vi "GenesysPS.destructor.vi"(0 "i ref in":refnum<vi>, 5 "error in (no error)":errorcluster) -> (19 "error out":errorcluster)   [LabVIEW 2014, in "GenesysPS.lvlib"]
doc: "This is the destructor of a class.\n\nLicense Agreement for this software:\n\nCopyright (C)\nGesellschaft für Schwerionenforschung, GSI\nPlanckstr. 1\n64291 Darmstadt\nGermany\n\nContact: D.Beck@gsi.de \n\nThis program is free software; you can redistribute it and/or modify it under the terms of the \nGNU General Public License as published by the Free Software Foundation; either version 2 of \nthe license, or (at your option) any later version.\n\nThis program is distributed in the hope that it will be useful, but WITHOUT ANY WARRANTY; \nwithout even the implied warranty of MERCHANTABILITY or FITNESS FOR A PARTICULAR PURPOSE. See the GNU General License for more details (http://www.gnu.org).\n\nGesellschaft für Schwerionenforschung, GSI\nPlanckstr. 1, 64291 Darmstadt, Germany\nFor all questions and ideas contact: M.Richter@gsi.de, H.Brand@gsi.de or D.Beck@gsi.de.\nLast update: 16-JUN-2004"
uses:
  GenesysPS.lvlib
  DIMPowerSupply/DIMPowerSupply.lvlib
  CSlibraries-extern/DimLVEvent/LVDimInterface/LVDimInterface.lvlib
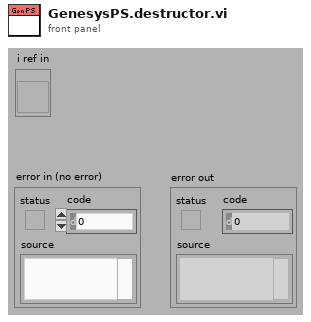
[diagram p1: front panel]
types:
  T1 = typedef "GenesysPS.lvlib/GenesysPS.i attribute.ctl" = cluster{"VISA name/ Heizinger":refnum<visa-resource-name>, "GEN Addr":i32, "WithTempInt?":bool, "TempLimit":dbl, "TemperatureID":i32, "Temp queue":refnum<queue>}
  T2 = enum16{"SetAttribute", "GetAttribute", "CreateAttribute", "DestroyAttribute", "DestroyAllAtributes"}
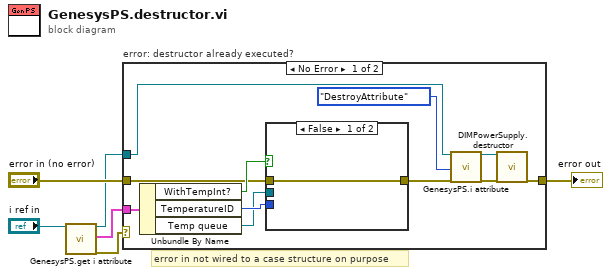
[diagram p0: block diagram]
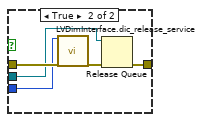
[diagram p2: hidden frame]
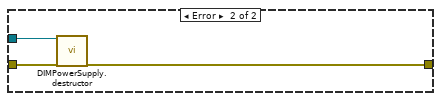
[diagram p3: hidden frame]
diagram:
  # "error in not wired to a case structure on purpose"
  n1 = call "GenesysPS.get i attribute.vi"("i ref in"="i ref in") -> ("i ref out"=w2:refnum<vi>, "i attribute"=w1:T1, "error out"=w3:errorcluster)  [unwired: 16 in]
  n2 = case "error: destructor already executed?" shown="No Error" w3 {
    tunnel: [w14 w24] -> w6
    tunnel: "error in (no error)" -> [w9 w25]
    tunnel: w2 -> [w13 w26]
    tunnel: w1 -> [w12 _]
    frame No Error {
      n3 = Unbundle By Name(w12) -> ("WithTempInt?"=w11:bool, "TemperatureID"=w8:i32, "Temp queue"=w7:refnum<queue>)
      n4 = case shown="False" w11 {
        tunnel: [w18 w21] -> w10
        tunnel: w9 -> [w18 w23]
        tunnel: w8 -> [_ w20]
        tunnel: w7 -> [_ w19]
        frame False {
        }
        frame True {
          n5 = call "LVDimInterface.dic_release_service.vi"("callBackID"=w20, "error in (no error)"=w23) -> ("error out"=w22:errorcluster)  [unwired: 17 in]
          n6 = Release Queue(queue=w19, error in (no error)=w22) -> (error out=w21:errorcluster)  [unwired: 1 in, 2 out]
        }
      }
      n7 = call "GenesysPS.i attribute.vi"("VI Refnum"=w13, "Action"=T2."DestroyAttribute", "error in (no error)"=w10) -> ("VI Refnum out"=w16:refnum<vi>, "error out"=w15:errorcluster)  [unwired: 14 in, 1 out]
      n8 = call "DIMPowerSupply.destructor.vi"("i ref in"=w16, "error in (no error)"=w15) -> ("error out"=w14:errorcluster)  [unwired: 17 in]
    }
    frame Error {
      n9 = call "DIMPowerSupply.destructor.vi"("i ref in"=w26, "error in (no error)"=w25) -> ("error out"=w24:errorcluster)  [unwired: 17 in]
    }
  }
  "error out" <- w6
